vi "Add Path Segment.vi"(10 "Path Segment":string, 11 "URI in":refnum<class "URI.lvclass">) -> (3 "URI out":refnum<class "URI.lvclass">)   [LabVIEW 2020, in "URI.lvlib" / "URI.lvclass"]
uses:
  URI.lvclass
  URI.lvclass/URI.ctl
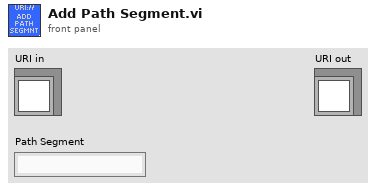
[diagram p1: front panel]
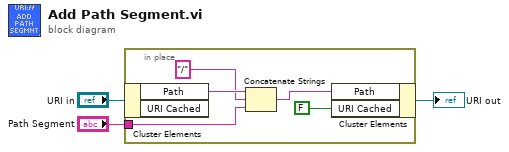
[diagram p0: block diagram]
diagram:
  n1 = in-place {
    in-place-border: "Path Segment" -> [w6]
    n2 = in-place-cluster #1("URI in") -> ("Path"=w8:string)  [unwired: 1 out]
    n3 = Concatenate Strings(w8, "/", w6) -> (w5:string)
    n4 = in-place-cluster #1("Path"=w5, "URI Cached"=FALSE ("String Cached")) -> (→"URI out":refnum<class "URI.lvclass">)
  }
